vi "Receive.vi"(8 "error in":errorcluster, 11 "framework in":refnum<class "Framework.lvclass">) -> (0 "error out":errorcluster, 3 "framework out":refnum<class "Framework.lvclass">)   [LabVIEW 2021, in "DSF Core.lvlib" / "Framework.lvclass"]
uses:
  Framework.lvclass
  Framework States.ctl
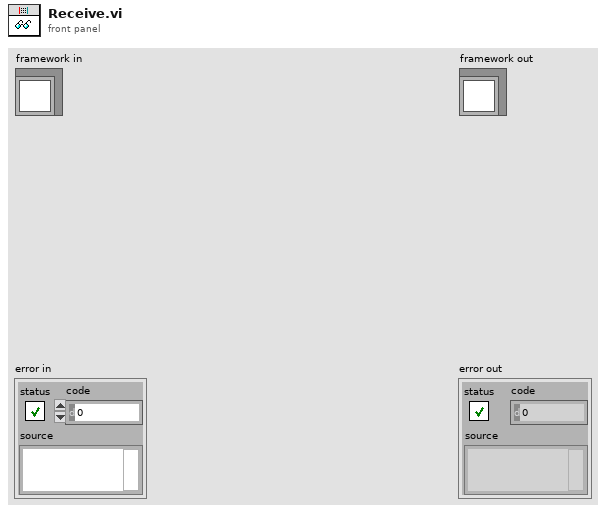
[diagram p1: front panel]
types:
  T1 = typedef "DSF Core.lvlib/Framework.lvclass/Framework States.ctl" = enum8{"Uninitialized", "Initialized", "Start", "Rx", "Tx", "Shutdown"}
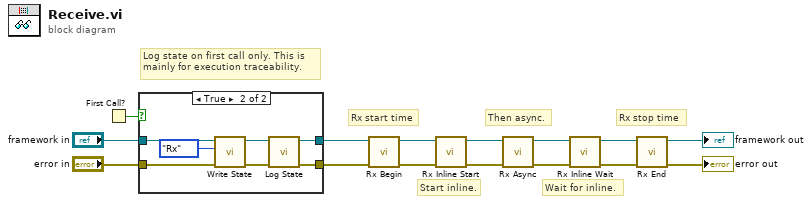
[diagram p0: block diagram]
diagram:
  # "Rx stop time"
  # "Rx start time"
  # "Log state on first call only. This is mainly for execution traceability."
  # "Wait for inline."
  # "Start inline."
  # "Then async."
  n1 = First Call?() -> (First Call?: T/F=w7:bool)
  n2 = case shown="True" w7 {
    tunnel: "error in" -> [w16 w21]
    tunnel: "framework in" -> [w17 w20]
    tunnel: [w16 w19] -> w9
    tunnel: [w17 w18] -> w8
    frame False {
    }
    frame True {
      n3 = call "Write State.vi"("error in (no error)"=w21, "state"=Framework_States."Rx", "Framework in"=w20) -> ("error out"=w22:errorcluster, "Framework out"=w23:refnum<class "Framework.lvclass">)  [unwired: 7 in]
      n4 = call "Log State.vi"("error in (no error)"=w22, "Framework in"=w23) -> ("error out"=w19:errorcluster, "Framework out"=w18:refnum<class "Framework.lvclass">)  [unwired: 8 in]
    }
  }
  n5 = call "Rx Begin.vi"("error in (no error)"=w9, "Framework in"=w8) -> ("error out"=w5:errorcluster, "Framework out"=w6:refnum<class "Framework.lvclass">)  [unwired: 8 in]
  n6 = call "Rx Inline Start.vi"("error in (no error)"=w5, "Framework in"=w6) -> ("error out"=w3:errorcluster, "Framework out"=w4:refnum<class "Framework.lvclass">)  [unwired: 8 in]
  n7 = call "Rx Async.vi"("error in (no error)"=w3, "Framework in"=w4) -> ("error out"=w1:errorcluster, "Framework out"=w2:refnum<class "Framework.lvclass">)  [unwired: 8 in]
  n8 = call "Rx Inline Wait.vi"("error in (no error)"=w1, "Framework in"=w2) -> ("error out"=w13:errorcluster, "Framework out"=w12:refnum<class "Framework.lvclass">)  [unwired: 8 in]
  n9 = call "Rx End.vi"("error in (no error)"=w13, "Framework in"=w12) -> ("error out"=→"error out":errorcluster, "Framework out"=→"framework out":refnum<class "Framework.lvclass">)  [unwired: 8 in]
